vi "Read Joystick.vi"(8 "Joystick Deadbanded Value (default of 0.1)":dbl, 10 "Joystick R 2 DevRef":T1, 11 "Joystick L 1 DevRef":T1) -> (0 "Wheel Lock":bool=TRUE, 1 "Joystick R 2 X Axis":dbl, 2 "Joystick L 1 Y Axis":dbl, 3 "Joystick L 1 X Axis":dbl, 4 "Radial Spin":bool, 5 "Revolver":bool)   [LabVIEW 2012]
uses:
  <vilib>/Rock Robotics/WPI/Joystick/WPI_JoystickDevRef.ctl
  <vilib>/Rock Robotics/WPI/Joystick/WPI_JoystickDeviceEnum.ctl
  Begin/Global Variables.vi
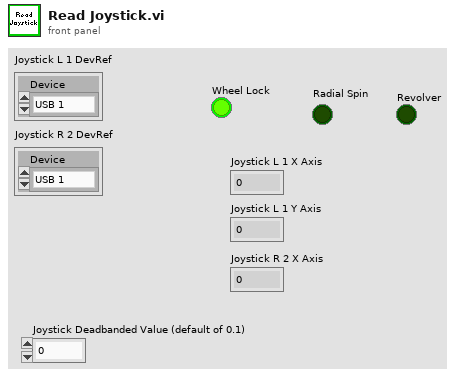
[diagram p1: front panel]
types:
  T1 = typedef "WPI_JoystickDevRef.ctl" = cluster{"Device":T2}
  T2 = typedef "WPI_JoystickDeviceEnum.ctl" = enum16{"USB 1", "USB 2", "USB 3", "USB 4", "Kinect 1", "Kinect 2"}
  T3 = typedef "WPI_JoystickButtonState.ctl" = cluster{"Button 1":bool, "Button 2":bool, "Button 3":bool, "Button 4":bool, "Button 5":bool, "Button 6":bool, "Button 7":bool, "Button 8":bool, "Button 9":bool, "Button 10":bool, "Button 11":bool, "Button 12":bool}
  T4 = cluster{"axis 1 (x)":dbl, "axis 2 (y)":dbl, "axis 3 (throttle)":dbl, "axis 4":dbl, "axis 5":dbl, "axis 6":dbl}
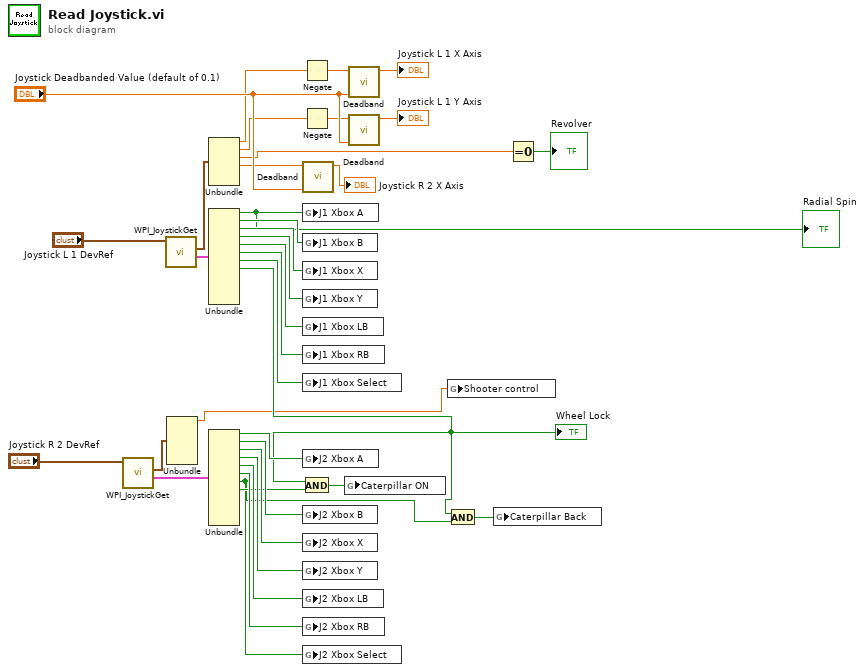
[diagram p0: block diagram]
diagram:
  n1 = call <vilib>:"WPI_JoystickGet.vi"("JoystickDevRef"="Joystick R 2 DevRef") -> ("Buttons"=w26:T3, "Axes"=w25:T4)  [unwired: 4 in, 1 out]
  n2 = call <vilib>:"WPI_JoystickGet.vi"("JoystickDevRef"="Joystick L 1 DevRef") -> ("Buttons"=w36:T3, "Axes"=w35:T4)  [unwired: 4 in, 1 out]
  n3 = Unbundle(w25) -> ("axis 1 (x)"=w3:dbl)  [unwired: 5 out]
  n4 = Unbundle(w35) -> ("axis 1 (x)"=w19:dbl, "axis 2 (y)"=w29:dbl, "axis 3 (throttle)"=w2:dbl, "axis 4"=w11:dbl)  [unwired: 2 out]
  n5 = Unbundle(w36) -> ("Button 1"=w4:bool, "Button 2"=w15:bool, "Button 3"=w21:bool, "Button 4"=w17:bool, "Button 5"=w27:bool, "Button 6"=w28:bool, "Button 7"=w9:bool, "Button 8"=w6:bool)  [unwired: 4 out]
  "Wheel Lock" <- w6
  "Radial Spin" <- w4
  n6 = Unbundle(w26) -> ("Button 1"=w23:bool, "Button 2"=w13:bool, "Button 3"=w16:bool, "Button 4"=w14:bool, "Button 5"=w22:bool, "Button 6"=w12:bool, "Button 7"=w5:bool, "Button 8"=w8:bool)  [unwired: 4 out]
  n7 = Negate(x=w19) -> (-x=w20:dbl)
  n8 = Negate(x=w29) -> (-x=w18:dbl)
  n9 = And(x=w6, y=w8) -> (x .and. y?=w10:bool)
  n10 = call "Deadband.vi"("Value to Deadband (default of 0.1)"="Joystick Deadbanded Value (default of 0.1)", "Value"=w11) -> ("Deadbanded Value"=→"Joystick R 2 X Axis":dbl)  [unwired: 9 in]
  n11 = global write "Global Variables.vi" "J1 Xbox A"(w4) -> ()
  n12 = global write "Global Variables.vi" "J1 Xbox B"(w15) -> ()
  n13 = global write "Global Variables.vi" "J1 Xbox X"(w21) -> ()
  n14 = global write "Global Variables.vi" "J1 Xbox Y"(w17) -> ()
  n15 = global write "Global Variables.vi" "J1 Xbox LB"(w27) -> ()
  n16 = global write "Global Variables.vi" "J1 Xbox RB"(w28) -> ()
  n17 = global write "Global Variables.vi" "J1 Xbox Select"(w9) -> ()
  n18 = global write "Global Variables.vi" "J2 Xbox A"(w23) -> ()
  n19 = global write "Global Variables.vi" "J2 Xbox B"(w13) -> ()
  n20 = global write "Global Variables.vi" "J2 Xbox X"(w16) -> ()
  n21 = global write "Global Variables.vi" "J2 Xbox Y"(w14) -> ()
  n22 = global write "Global Variables.vi" "J2 Xbox LB"(w22) -> ()
  n23 = global write "Global Variables.vi" "J2 Xbox RB"(w12) -> ()
  n24 = global write "Global Variables.vi" "J2 Xbox Select"(w5) -> ()
  n25 = global write "Global Variables.vi" "Caterpillar ON"(w10) -> ()
  n26 = call "Deadband.vi"("Value to Deadband (default of 0.1)"="Joystick Deadbanded Value (default of 0.1)", "Value"=w20) -> ("Deadbanded Value"=→"Joystick L 1 X Axis":dbl)  [unwired: 9 in]
  n27 = call "Deadband.vi"("Value to Deadband (default of 0.1)"="Joystick Deadbanded Value (default of 0.1)", "Value"=w18) -> ("Deadbanded Value"=→"Joystick L 1 Y Axis":dbl)  [unwired: 9 in]
  n28 = global write "Global Variables.vi" "Shooter control"(w3) -> ()
  n29 = And(x=w6, y=w5) -> (x .and. y?=w7:bool)
  n30 = global write "Global Variables.vi" "Caterpillar Back"(w7) -> ()
  n31 = Equal To 0?(x=w2) -> (x = 0?=→"Revolver":bool)
